vi "Multiply-gain.vi"(10 "State (X)":dbl[](array[numeric]), 11 "Gain (K)":dbl[](array[numeric])) -> (2 "Kx":dbl)   [LabVIEW 2016]
uses:
  <vilib>/Analysis/baseanly.llb/Real Dot Product.vi
  <vilib>/Analysis/NI_AALBase.lvlib
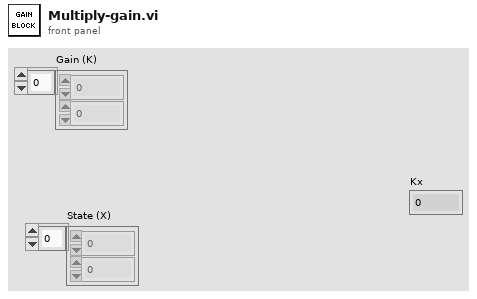
[diagram p1: front panel]
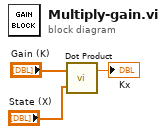
[diagram p0: block diagram]
diagram:
  n1 = call-poly <vilib>:"Dot Product.vi"("Y Vector"="State (X)", "X Vector"="Gain (K)") -> ("X * Y"=→"Kx":dbl)  [unwired: 1 out]
